vi "Autonomous Independent.vi"() -> ()   [LabVIEW 2015]
doc: "This VI is called when autonomous begins, and will automatically be terminated when autonomous ends. You can carry out timed or sensor driven robot movement independently without needing to return to the caller."
uses:
  Robot Global Data.vi
  <vilib>/Rock Robotics/Network Tables/NT Read Number.vi
panel:
  out "Speed":dbl
  out "Stuck?":bool
  out "Position":dbl
  out "Temporary Center":dbl
  # "Be sure to right-click and choose Data Operations>>Make Current Value default if you want to save the array values with the VI"
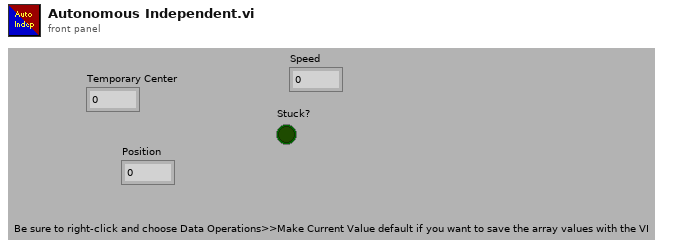
[diagram p1: front panel]
types:
  T1 = typedef "Relevant Data.ctl" = cluster{"Area":dbl, "CH Area":dbl, "BR Width":dbl, "BR Height":dbl, "BR Left":dbl, "BR Right":dbl}
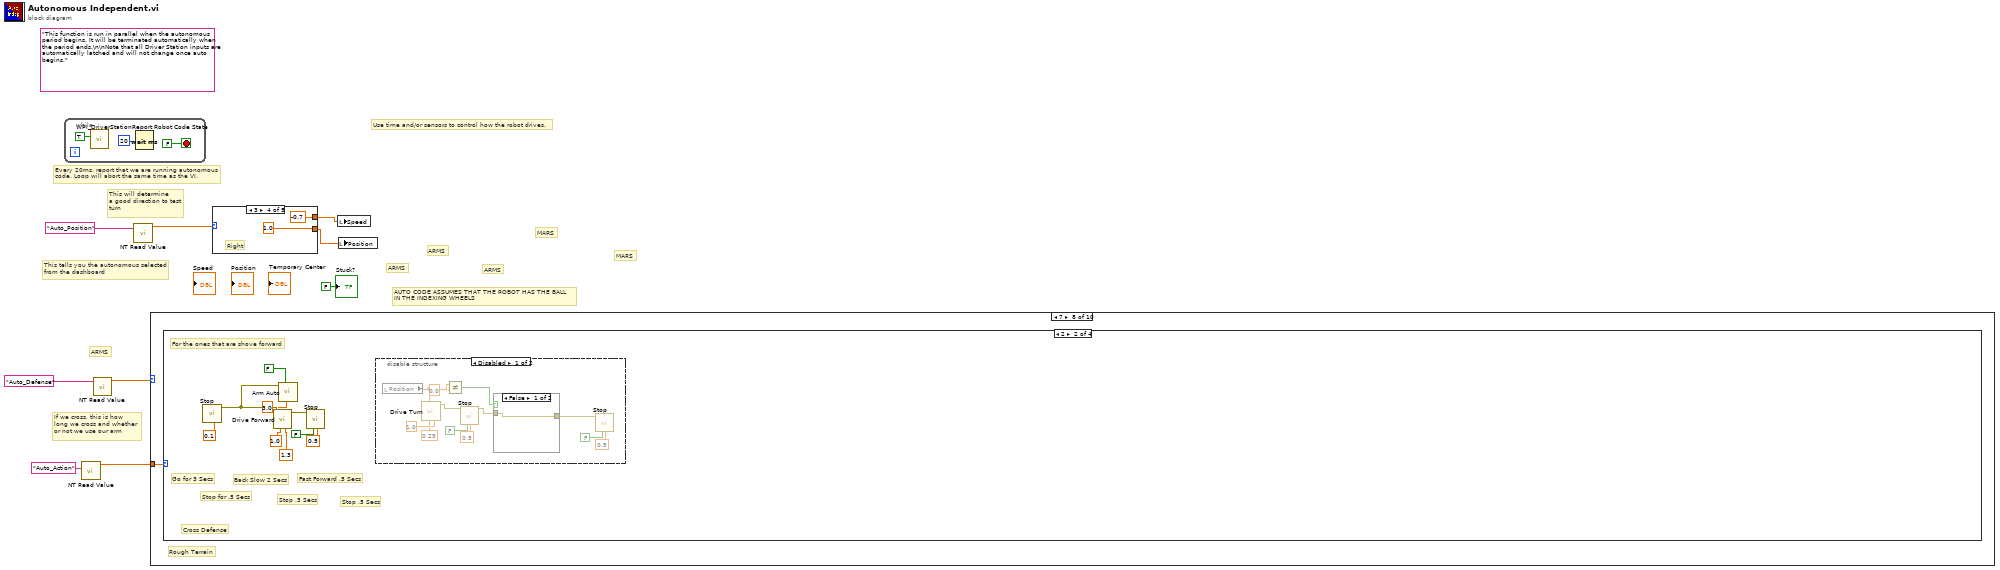
[diagram p0: block diagram]
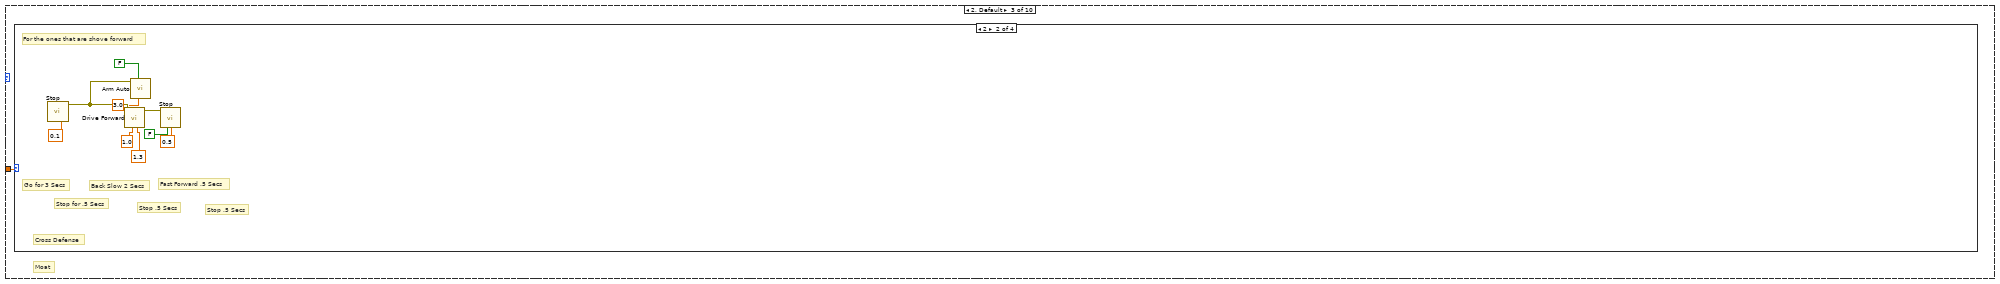
[diagram p4: hidden frame]
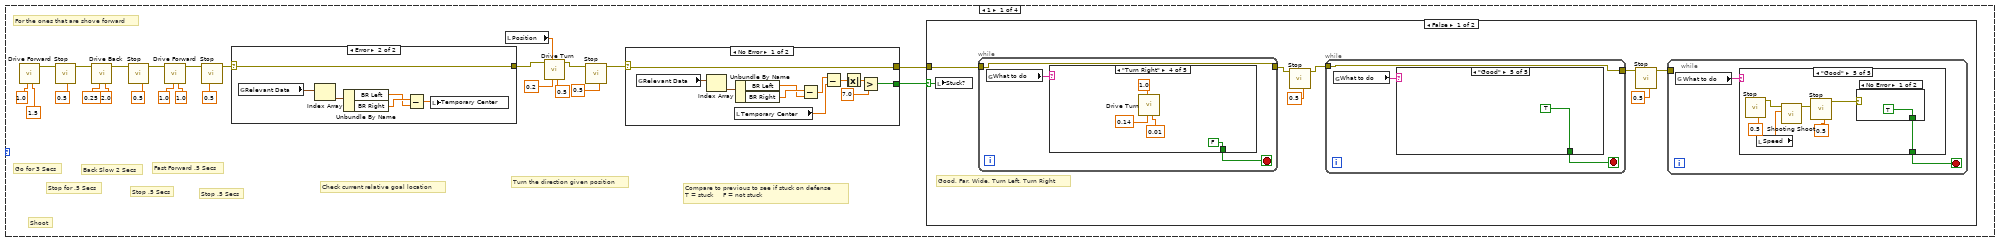
[diagram p5: hidden frame]
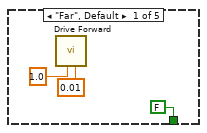
[diagram p6: hidden frame]
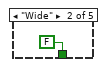
[diagram p7: hidden frame]
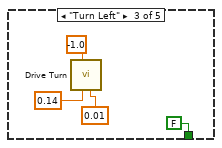
[diagram p8: hidden frame]
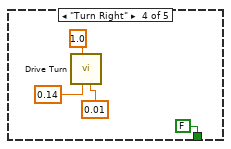
[diagram p9: hidden frame]
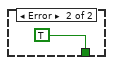
[diagram p10: hidden frame]
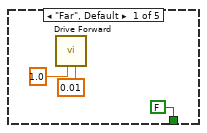
[diagram p11: hidden frame]
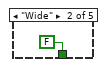
[diagram p12: hidden frame]
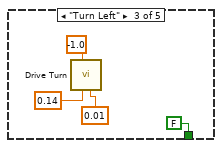
[diagram p13: hidden frame]
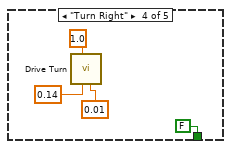
[diagram p14: hidden frame]
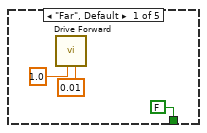
[diagram p15: hidden frame]
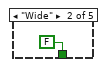
[diagram p16: hidden frame]
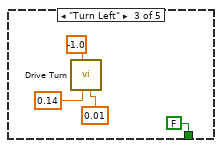
[diagram p17: hidden frame]
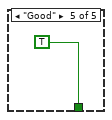
[diagram p18: hidden frame]
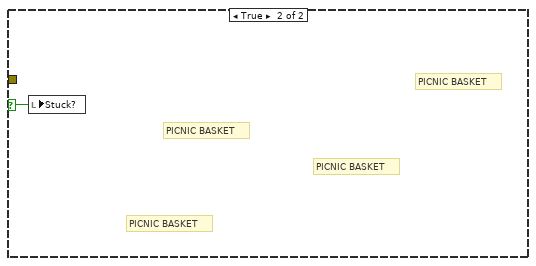
[diagram p19: hidden frame]
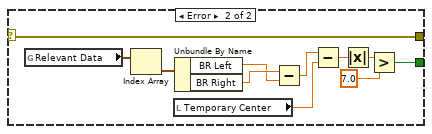
[diagram p20: hidden frame]
diagram:
  (unwired) "This function is run in parallel when the autonomous period begins. It will be terminated automatically when the period ends.\n\nNote that all Driver Station inputs are automatically latched and will not change once auto begins."
  # "MARS"
  # "MARS"
  # "ARMS"
  # "ARMS"
  # "ARMS"
  # "ARMS"
  # "AUTO CODE ASSUMES THAT THE ROBOT HAS THE BALL\nIN THE INDEXING WHEELS"
  # "If we cross, this is how\nlong we cross and whether \nor not we use our arm"
  # "This will determine\na good direction to test\nturn"
  # "This tells you the autonomous selected\nfrom the dashboard"
  # "Every 20ms, report that we are running autonomous\ncode. Loop will abort the same time as the VI."
  # "Use time and/or sensors to control how the robot drives."
  n1 = while {
    stop <- FALSE stop-if-true
    n2 = call <vilib>:"WPI_DriverStationReport Robot Code State.vi"("Autonomous"=TRUE) -> ()  [unwired: 10 in, 1 out]
    n3 = Wait (ms)(milliseconds to wait=u32 20) -> ()  [unwired: 1 out]
  }
  n4 = call-poly <vilib>:"NT Read Value.vi"("Name"="Auto_Action") -> ("Numeric"=w2:dbl)  [unwired: 9 in, 1 out]
  n5 = call-poly <vilib>:"NT Read Value.vi"("Name"="Auto_Defense") -> ("Numeric"=w7:dbl)  [unwired: 9 in, 1 out]
  n6 = call-poly <vilib>:"NT Read Value.vi"("Name"="Auto_Position") -> ("Numeric"=w8:dbl)  [unwired: 9 in, 1 out]
  n7 = case shown="7" w7 {
    tunnel: w2 -> [_ _ w13 w150 _ _ w287 w424 _ w579]
    frame 0 {
      # "Portcullis"
    }
    frame 1 {
      # "Cheval de Frise"
    }
    frame 2, Default {
      # "Moat"
      n8 = case shown="2" w13 {
        frame 1 {
          # "Shoot"
          # "Check current relative goal location"
          # "Stop .5 Secs"
          # "Turn the direction given position"
          # "Compare to previous to see if stuck on defense\nT = stuck     F = not stuck"
          # "Fast Forward .5 Secs"
          # "Stop .5 Secs"
          # "Back Slow 2 Secs"
          # "Stop for .5 Secs"
          # "Go for 3 Secs"
          # "For the ones that are shove forward"
          n9 = call "Drive Forward.vi"("Time"=1.5, "Speed"=1.0) -> ("error out"=w37:errorcluster)  [unwired: 9 in]
          n10 = call "Stop.vi"("Time"=0.5, "error in"=w37) -> ("error out"=w36:errorcluster)  [unwired: 8 in, 1 out]
          n11 = call "Drive Back.vi"("Time"=2.0, "Speed"=0.25, "error in"=w36) -> ("error out"=w35:errorcluster)  [unwired: 8 in]
          n12 = call "Stop.vi"("Time"=0.5, "error in"=w35) -> ("error out"=w34:errorcluster)  [unwired: 8 in, 1 out]
          n13 = call "Drive Forward.vi"("Time"=1.0, "Speed"=1.0, "error in"=w34) -> ("error out"=w33:errorcluster)  [unwired: 8 in]
          n14 = call "Stop.vi"("Time"=0.5, "error in"=w33) -> ("error out"=w23:errorcluster)  [unwired: 8 in, 1 out]
          n15 = case shown="Error" w23 {
            selector: w23 -> [w124 w130]
            tunnel: [w124 w130] -> w22
            frame No Error {
              n16 = global read "Robot Global Data.vi" "Relevant Data"() -> (w129:T1[])
              n17 = Index Array(array=w129) -> (element=w128:T1)  [unwired: 1 in]
              n18 = Unbundle By Name(w128) -> ("BR Left"=w126:dbl, "BR Right"=w127:dbl)
              n19 = Subtract(x=w127, y=w126) -> (x-y=w125:dbl)
              n20 = local write "Temporary Center"(w125) -> ()
            }
            frame Error {
              n21 = global read "Robot Global Data.vi" "Relevant Data"() -> (w135:T1[])
              n22 = Index Array(array=w135) -> (element=w134:T1)  [unwired: 1 in]
              n23 = Unbundle By Name(w134) -> ("BR Left"=w132:dbl, "BR Right"=w133:dbl)
              n24 = Subtract(x=w133, y=w132) -> (x-y=w131:dbl)
              n25 = local write "Temporary Center"(w131) -> ()
            }
          }
          n26 = local read "Position"() -> (w21:dbl)
          n27 = call "Drive Turn.vi"("Time"=0.5, "Speed"=0.2, "Direction"=w21, "error in"=w22) -> ("error out"=w17:errorcluster)  [unwired: 7 in]
          n28 = call "Stop.vi"("Time"=0.5, "error in"=w17) -> ("error out"=w16:errorcluster)  [unwired: 8 in, 1 out]
          n29 = case shown="No Error" w16 {
            selector: w16 -> [w108 w119]
            tunnel: [w108 w119] -> w14
            tunnel: [w102 w113] -> w18
            frame No Error {
              n30 = global read "Robot Global Data.vi" "Relevant Data"() -> (w112:T1[])
              n31 = Index Array(array=w112) -> (element=w111:T1)  [unwired: 1 in]
              n32 = local read "Temporary Center"() -> (w106:dbl)
              n33 = Unbundle By Name(w111) -> ("BR Left"=w109:dbl, "BR Right"=w110:dbl)
              n34 = Subtract(x=w110, y=w109) -> (x-y=w107:dbl)
              n35 = Subtract(x=w107, y=w106) -> (x-y=w105:dbl)
              n36 = Absolute Value(x=w105) -> (abs(x)=w104:dbl)
              n37 = Greater?(x=w104, y=7.0) -> (0:w102:bool)
            }
            frame Error {
              n38 = global read "Robot Global Data.vi" "Relevant Data"() -> (w123:T1[])
              n39 = Index Array(array=w123) -> (element=w122:T1)  [unwired: 1 in]
              n40 = local read "Temporary Center"() -> (w117:dbl)
              n41 = Unbundle By Name(w122) -> ("BR Left"=w120:dbl, "BR Right"=w121:dbl)
              n42 = Subtract(x=w121, y=w120) -> (x-y=w118:dbl)
              n43 = Subtract(x=w118, y=w117) -> (x-y=w116:dbl)
              n44 = Absolute Value(x=w116) -> (abs(x)=w115:dbl)
              n45 = Greater?(x=w115, y=7.0) -> (0:w113:bool)
            }
          }
          n46 = case shown="False" w18 {
            selector: w18 -> [w45 w101]
            tunnel: w14 -> [w44 _]
            frame False {
              # "Good, Far, Wide, Turn Left, Turn Right"
              n47 = local write "Stuck?"(w45) -> ()
              n48 = while {
                tunnel: w44 -> [w85]
                tunnel: [w85] -> w43
                stop <- w86 stop-if-true
                n49 = global read "Robot Global Data.vi" "What to do"() -> (w87:string)
                n50 = case shown="\"Turn Right\"" w87 {
                  tunnel: [FALSE FALSE FALSE FALSE TRUE] -> w86
                  frame "Far", Default {
                    n51 = call "Drive Forward.vi"("Time"=0.01, "Speed"=1.0) -> ()  [unwired: 9 in, 1 out]
                  }
                  frame "Wide" {
                  }
                  frame "Turn Left" {
                    n52 = call "Drive Turn.vi"("Time"=0.01, "Speed"=0.14, "Direction"=-1.0) -> ()  [unwired: 8 in, 1 out]
                  }
                  frame "Turn Right" {
                    n53 = call "Drive Turn.vi"("Time"=0.01, "Speed"=0.14, "Direction"=1.0) -> ()  [unwired: 8 in, 1 out]
                  }
                  frame "Good" {
                  }
                }
              }
              n54 = call "Stop.vi"("Time"=0.5, "error in"=w43) -> ("error out"=w42:errorcluster)  [unwired: 8 in, 1 out]
              n55 = while {
                tunnel: w42 -> [w69]
                tunnel: [w69] -> w40
                stop <- w70 stop-if-true
                n56 = global read "Robot Global Data.vi" "What to do"() -> (w71:string)
                n57 = case shown="\"Good\"" w71 {
                  tunnel: [FALSE FALSE FALSE FALSE TRUE] -> w70
                  frame "Far", Default {
                    n58 = call "Drive Forward.vi"("Time"=0.01, "Speed"=1.0) -> ()  [unwired: 9 in, 1 out]
                  }
                  frame "Wide" {
                  }
                  frame "Turn Left" {
                    n59 = call "Drive Turn.vi"("Time"=0.01, "Speed"=0.14, "Direction"=-1.0) -> ()  [unwired: 8 in, 1 out]
                  }
                  frame "Turn Right" {
                    n60 = call "Drive Turn.vi"("Time"=0.01, "Speed"=0.14, "Direction"=1.0) -> ()  [unwired: 8 in, 1 out]
                  }
                  frame "Good" {
                  }
                }
              }
              n61 = call "Stop.vi"("Time"=0.5, "error in"=w40) -> ("error out"=w39:errorcluster)  [unwired: 8 in, 1 out]
              n62 = while {
                tunnel: w39 -> [_]
                stop <- w46 stop-if-true
                n63 = global read "Robot Global Data.vi" "What to do"() -> (w47:string)
                n64 = case shown="\"Good\"" w47 {
                  tunnel: [FALSE FALSE FALSE FALSE w64] -> w46
                  frame "Far", Default {
                    n65 = call "Drive Forward.vi"("Time"=0.01, "Speed"=1.0) -> ()  [unwired: 9 in, 1 out]
                  }
                  frame "Wide" {
                  }
                  frame "Turn Left" {
                    n66 = call "Drive Turn.vi"("Time"=0.01, "Speed"=0.14, "Direction"=-1.0) -> ()  [unwired: 8 in, 1 out]
                  }
                  frame "Turn Right" {
                    n67 = call "Drive Turn.vi"("Time"=0.01, "Speed"=0.14, "Direction"=1.0) -> ()  [unwired: 8 in, 1 out]
                  }
                  frame "Good" {
                    n68 = call "Stop.vi"("Time"=0.5) -> ("error out"=w61:errorcluster)  [unwired: 9 in, 1 out]
                    n69 = local read "Speed"() -> (w60:dbl)
                    n70 = call "Shooting Shoot.vi"("Power"=w60, "error in (no error)"=w61) -> ("error out"=w62:errorcluster)  [unwired: 9 in]
                    n71 = call "Stop.vi"("Time"=0.5, "error in"=w62) -> ("error out"=w65:errorcluster)  [unwired: 8 in, 1 out]
                    n72 = case shown="No Error" w65 {
                      tunnel: [TRUE TRUE] -> w64
                      frame No Error {
                      }
                      frame Error {
                      }
                    }
                  }
                }
              }
            }
            frame True {
              # "PICNIC BASKET"
              # "PICNIC BASKET"
              # "PICNIC BASKET"
              # "PICNIC BASKET"
              n73 = local write "Stuck?"(w101) -> ()
            }
          }
        }
        frame 2 {
          # "Cross Defense"
          # "Stop .5 Secs"
          # "Fast Forward .5 Secs"
          # "Stop .5 Secs"
          # "Back Slow 2 Secs"
          # "Stop for .5 Secs"
          # "Go for 3 Secs"
          # "For the ones that are shove forward"
          n74 = call "Stop.vi"("Time"=0.1) -> ("error out"=w139:errorcluster)  [unwired: 9 in, 1 out]
          n75 = call "Drive Forward.vi"("Time"=1.3, "Speed"=1.0, "error in"=w139) -> ("error out"=w144:errorcluster)  [unwired: 8 in]
          n76 = call "Arm Auto.vi"("Time"=3.0, "U=T\nD=F"=FALSE ("U=T\nD=F"), "error in"=w139) -> ()  [unwired: 8 in, 1 out]
          n77 = call "Stop.vi"("Time"=0.5, "Stop Arm?"=FALSE, "error in"=w144) -> ()  [unwired: 7 in, 2 out]
        }
        frame 3 {
          # "Up to Line"
          # "Stop for .5 Secs"
          # "Go for 3 Secs"
          # "For the ones that are shove forward"
          n78 = call "Drive Forward.vi"("Time"=0.5, "Speed"=1.0) -> ("error out"=w148:errorcluster)  [unwired: 9 in]
          n79 = call "Stop.vi"("Time"=0.5, "error in"=w148) -> ()  [unwired: 8 in, 2 out]
        }
        frame 0, Default {
          # "Disabled"
          n80 = call "Stop.vi"("Time"=0.5) -> ()  [unwired: 9 in, 2 out]
        }
      }
    }
    frame 3 {
      # "Ramparts"
      n81 = case shown="2" w150 {
        frame 1 {
          # "Shoot"
          # "Check current relative goal location"
          # "Stop .5 Secs"
          # "Turn the direction given position"
          # "Compare to previous to see if stuck on defense\nT = stuck     F = not stuck"
          # "Fast Forward .5 Secs"
          # "Stop .5 Secs"
          # "Back Slow 2 Secs"
          # "Stop for .5 Secs"
          # "Go for 3 Secs"
          # "For the ones that are shove forward"
          n82 = call "Drive Forward.vi"("Time"=1.5, "Speed"=1.0) -> ("error out"=w174:errorcluster)  [unwired: 9 in]
          n83 = call "Stop.vi"("Time"=0.5, "error in"=w174) -> ("error out"=w173:errorcluster)  [unwired: 8 in, 1 out]
          n84 = call "Drive Back.vi"("Time"=2.0, "Speed"=0.25, "error in"=w173) -> ("error out"=w172:errorcluster)  [unwired: 8 in]
          n85 = call "Stop.vi"("Time"=0.5, "error in"=w172) -> ("error out"=w171:errorcluster)  [unwired: 8 in, 1 out]
          n86 = call "Drive Forward.vi"("Time"=1.0, "Speed"=1.0, "error in"=w171) -> ("error out"=w170:errorcluster)  [unwired: 8 in]
          n87 = call "Stop.vi"("Time"=0.5, "error in"=w170) -> ("error out"=w160:errorcluster)  [unwired: 8 in, 1 out]
          n88 = case shown="Error" w160 {
            selector: w160 -> [w261 w267]
            tunnel: [w261 w267] -> w159
            frame No Error {
              n89 = global read "Robot Global Data.vi" "Relevant Data"() -> (w266:T1[])
              n90 = Index Array(array=w266) -> (element=w265:T1)  [unwired: 1 in]
              n91 = Unbundle By Name(w265) -> ("BR Left"=w263:dbl, "BR Right"=w264:dbl)
              n92 = Subtract(x=w264, y=w263) -> (x-y=w262:dbl)
              n93 = local write "Temporary Center"(w262) -> ()
            }
            frame Error {
              n94 = global read "Robot Global Data.vi" "Relevant Data"() -> (w272:T1[])
              n95 = Index Array(array=w272) -> (element=w271:T1)  [unwired: 1 in]
              n96 = Unbundle By Name(w271) -> ("BR Left"=w269:dbl, "BR Right"=w270:dbl)
              n97 = Subtract(x=w270, y=w269) -> (x-y=w268:dbl)
              n98 = local write "Temporary Center"(w268) -> ()
            }
          }
          n99 = call "Drive Turn.vi"("Time"=0.5, "Speed"=0.2, "Direction"=-1.0, "error in"=w159) -> ("error out"=w155:errorcluster)  [unwired: 7 in]
          n100 = call "Stop.vi"("Time"=0.5, "error in"=w155) -> ("error out"=w154:errorcluster)  [unwired: 8 in, 1 out]
          n101 = case shown="No Error" w154 {
            selector: w154 -> [w245 w256]
            tunnel: [w245 w256] -> w152
            tunnel: [w239 w250] -> w156
            frame No Error {
              n102 = global read "Robot Global Data.vi" "Relevant Data"() -> (w249:T1[])
              n103 = Index Array(array=w249) -> (element=w248:T1)  [unwired: 1 in]
              n104 = local read "Temporary Center"() -> (w243:dbl)
              n105 = Unbundle By Name(w248) -> ("BR Left"=w246:dbl, "BR Right"=w247:dbl)
              n106 = Subtract(x=w247, y=w246) -> (x-y=w244:dbl)
              n107 = Subtract(x=w244, y=w243) -> (x-y=w242:dbl)
              n108 = Absolute Value(x=w242) -> (abs(x)=w241:dbl)
              n109 = Greater?(x=w241, y=7.0) -> (0:w239:bool)
            }
            frame Error {
              n110 = global read "Robot Global Data.vi" "Relevant Data"() -> (w260:T1[])
              n111 = Index Array(array=w260) -> (element=w259:T1)  [unwired: 1 in]
              n112 = local read "Temporary Center"() -> (w254:dbl)
              n113 = Unbundle By Name(w259) -> ("BR Left"=w257:dbl, "BR Right"=w258:dbl)
              n114 = Subtract(x=w258, y=w257) -> (x-y=w255:dbl)
              n115 = Subtract(x=w255, y=w254) -> (x-y=w253:dbl)
              n116 = Absolute Value(x=w253) -> (abs(x)=w252:dbl)
              n117 = Greater?(x=w252, y=7.0) -> (0:w250:bool)
            }
          }
          n118 = case shown="False" w156 {
            selector: w156 -> [w182 w238]
            tunnel: w152 -> [w181 _]
            frame False {
              # "Good, Far, Wide, Turn Left, Turn Right"
              n119 = local write "Stuck?"(w182) -> ()
              n120 = while {
                tunnel: w181 -> [w222]
                tunnel: [w222] -> w180
                stop <- w223 stop-if-true
                n121 = global read "Robot Global Data.vi" "What to do"() -> (w224:string)
                n122 = case shown="\"Turn Right\"" w224 {
                  tunnel: [FALSE FALSE FALSE FALSE TRUE] -> w223
                  frame "Far", Default {
                    n123 = call "Drive Forward.vi"("Time"=0.01, "Speed"=1.0) -> ()  [unwired: 9 in, 1 out]
                  }
                  frame "Wide" {
                  }
                  frame "Turn Left" {
                    n124 = call "Drive Turn.vi"("Time"=0.01, "Speed"=0.14, "Direction"=-1.0) -> ()  [unwired: 8 in, 1 out]
                  }
                  frame "Turn Right" {
                    n125 = call "Drive Turn.vi"("Time"=0.01, "Speed"=0.14, "Direction"=1.0) -> ()  [unwired: 8 in, 1 out]
                  }
                  frame "Good" {
                  }
                }
              }
              n126 = call "Stop.vi"("Time"=0.5, "error in"=w180) -> ("error out"=w179:errorcluster)  [unwired: 8 in, 1 out]
              n127 = while {
                tunnel: w179 -> [w206]
                tunnel: [w206] -> w177
                stop <- w207 stop-if-true
                n128 = global read "Robot Global Data.vi" "What to do"() -> (w208:string)
                n129 = case shown="\"Good\"" w208 {
                  tunnel: [FALSE FALSE FALSE FALSE TRUE] -> w207
                  frame "Far", Default {
                    n130 = call "Drive Forward.vi"("Time"=0.01, "Speed"=1.0) -> ()  [unwired: 9 in, 1 out]
                  }
                  frame "Wide" {
                  }
                  frame "Turn Left" {
                    n131 = call "Drive Turn.vi"("Time"=0.01, "Speed"=0.14, "Direction"=-1.0) -> ()  [unwired: 8 in, 1 out]
                  }
                  frame "Turn Right" {
                    n132 = call "Drive Turn.vi"("Time"=0.01, "Speed"=0.14, "Direction"=1.0) -> ()  [unwired: 8 in, 1 out]
                  }
                  frame "Good" {
                  }
                }
              }
              n133 = call "Stop.vi"("Time"=0.5, "error in"=w177) -> ("error out"=w176:errorcluster)  [unwired: 8 in, 1 out]
              n134 = while {
                tunnel: w176 -> [_]
                stop <- w183 stop-if-true
                n135 = global read "Robot Global Data.vi" "What to do"() -> (w184:string)
                n136 = case shown="\"Good\"" w184 {
                  tunnel: [FALSE FALSE FALSE FALSE w201] -> w183
                  frame "Far", Default {
                    n137 = call "Drive Forward.vi"("Time"=0.01, "Speed"=1.0) -> ()  [unwired: 9 in, 1 out]
                  }
                  frame "Wide" {
                  }
                  frame "Turn Left" {
                    n138 = call "Drive Turn.vi"("Time"=0.01, "Speed"=0.14, "Direction"=-1.0) -> ()  [unwired: 8 in, 1 out]
                  }
                  frame "Turn Right" {
                    n139 = call "Drive Turn.vi"("Time"=0.01, "Speed"=0.14, "Direction"=1.0) -> ()  [unwired: 8 in, 1 out]
                  }
                  frame "Good" {
                    n140 = call "Stop.vi"("Time"=0.5) -> ("error out"=w198:errorcluster)  [unwired: 9 in, 1 out]
                    n141 = local read "Speed"() -> (w197:dbl)
                    n142 = call "Shooting Shoot.vi"("Power"=w197, "error in (no error)"=w198) -> ("error out"=w199:errorcluster)  [unwired: 9 in]
                    n143 = call "Stop.vi"("Time"=0.5, "error in"=w199) -> ("error out"=w202:errorcluster)  [unwired: 8 in, 1 out]
                    n144 = case shown="No Error" w202 {
                      tunnel: [TRUE TRUE] -> w201
                      frame No Error {
                      }
                      frame Error {
                      }
                    }
                  }
                }
              }
            }
            frame True {
              # "PICNIC BASKET"
              # "PICNIC BASKET"
              # "PICNIC BASKET"
              # "PICNIC BASKET"
              n145 = local write "Stuck?"(w238) -> ()
            }
          }
        }
        frame 2 {
          # "Cross Defense"
          # "Stop .5 Secs"
          # "Fast Forward .5 Secs"
          # "Stop .5 Secs"
          # "Back Slow 2 Secs"
          # "Stop for .5 Secs"
          # "Go for 3 Secs"
          # "For the ones that are shove forward"
          n146 = call "Stop.vi"("Time"=0.1) -> ("error out"=w274:errorcluster)  [unwired: 9 in, 1 out]
          n147 = call "Drive Forward.vi"("Time"=1.3, "Speed"=1.0, "error in"=w274) -> ("error out"=w279:errorcluster)  [unwired: 8 in]
          n148 = call "Stop.vi"("Time"=0.5, "Stop Arm?"=FALSE, "error in"=w279) -> ()  [unwired: 7 in, 2 out]
        }
        frame 3 {
          # "Up to Line"
          # "Stop for .5 Secs"
          # "Go for 3 Secs"
          # "For the ones that are shove forward"
          n149 = call "Drive Forward.vi"("Time"=0.5, "Speed"=1.0) -> ("error out"=w283:errorcluster)  [unwired: 9 in]
          n150 = call "Stop.vi"("Time"=0.5, "error in"=w283) -> ()  [unwired: 8 in, 2 out]
        }
        frame 0, Default {
          # "Disabled"
          n151 = call "Stop.vi"("Time"=0.5) -> ()  [unwired: 9 in, 2 out]
        }
      }
    }
    frame 4 {
      # "Drawbridge"
      n152 = call "Stop.vi"("Time"=0.5) -> ()  [unwired: 9 in, 2 out]
    }
    frame 5 {
      # "Sally Port"
      n153 = call "Stop.vi"("Time"=0.5) -> ()  [unwired: 9 in, 2 out]
    }
    frame 6 {
      # "Rock Wall"
      n154 = case shown="2" w287 {
        frame 1 {
          # "Shoot"
          # "Check current relative goal location"
          # "Stop .5 Secs"
          # "Turn the direction given position"
          # "Compare to previous to see if stuck on defense\nT = stuck     F = not stuck"
          # "Fast Forward .5 Secs"
          # "Stop .5 Secs"
          # "Back Slow 2 Secs"
          # "Stop for .5 Secs"
          # "Go for 3 Secs"
          # "For the ones that are shove forward"
          n155 = call "Drive Forward.vi"("Time"=1.5, "Speed"=1.0) -> ("error out"=w311:errorcluster)  [unwired: 9 in]
          n156 = call "Stop.vi"("Time"=0.5, "error in"=w311) -> ("error out"=w310:errorcluster)  [unwired: 8 in, 1 out]
          n157 = call "Drive Back.vi"("Time"=2.0, "Speed"=0.25, "error in"=w310) -> ("error out"=w309:errorcluster)  [unwired: 8 in]
          n158 = call "Stop.vi"("Time"=0.5, "error in"=w309) -> ("error out"=w308:errorcluster)  [unwired: 8 in, 1 out]
          n159 = call "Drive Forward.vi"("Time"=1.0, "Speed"=1.0, "error in"=w308) -> ("error out"=w307:errorcluster)  [unwired: 8 in]
          n160 = call "Stop.vi"("Time"=0.5, "error in"=w307) -> ("error out"=w297:errorcluster)  [unwired: 8 in, 1 out]
          n161 = case shown="Error" w297 {
            selector: w297 -> [w398 w404]
            tunnel: [w398 w404] -> w296
            frame No Error {
              n162 = global read "Robot Global Data.vi" "Relevant Data"() -> (w403:T1[])
              n163 = Index Array(array=w403) -> (element=w402:T1)  [unwired: 1 in]
              n164 = Unbundle By Name(w402) -> ("BR Left"=w400:dbl, "BR Right"=w401:dbl)
              n165 = Subtract(x=w401, y=w400) -> (x-y=w399:dbl)
              n166 = local write "Temporary Center"(w399) -> ()
            }
            frame Error {
              n167 = global read "Robot Global Data.vi" "Relevant Data"() -> (w409:T1[])
              n168 = Index Array(array=w409) -> (element=w408:T1)  [unwired: 1 in]
              n169 = Unbundle By Name(w408) -> ("BR Left"=w406:dbl, "BR Right"=w407:dbl)
              n170 = Subtract(x=w407, y=w406) -> (x-y=w405:dbl)
              n171 = local write "Temporary Center"(w405) -> ()
            }
          }
          n172 = local read "Position"() -> (w295:dbl)
          n173 = call "Drive Turn.vi"("Time"=0.5, "Speed"=0.2, "Direction"=w295, "error in"=w296) -> ("error out"=w291:errorcluster)  [unwired: 7 in]
          n174 = call "Stop.vi"("Time"=0.5, "error in"=w291) -> ("error out"=w290:errorcluster)  [unwired: 8 in, 1 out]
          n175 = case shown="No Error" w290 {
            selector: w290 -> [w382 w393]
            tunnel: [w382 w393] -> w288
            tunnel: [w376 w387] -> w292
            frame No Error {
              n176 = global read "Robot Global Data.vi" "Relevant Data"() -> (w386:T1[])
              n177 = Index Array(array=w386) -> (element=w385:T1)  [unwired: 1 in]
              n178 = local read "Temporary Center"() -> (w380:dbl)
              n179 = Unbundle By Name(w385) -> ("BR Left"=w383:dbl, "BR Right"=w384:dbl)
              n180 = Subtract(x=w384, y=w383) -> (x-y=w381:dbl)
              n181 = Subtract(x=w381, y=w380) -> (x-y=w379:dbl)
              n182 = Absolute Value(x=w379) -> (abs(x)=w378:dbl)
              n183 = Greater?(x=w378, y=7.0) -> (0:w376:bool)
            }
            frame Error {
              n184 = global read "Robot Global Data.vi" "Relevant Data"() -> (w397:T1[])
              n185 = Index Array(array=w397) -> (element=w396:T1)  [unwired: 1 in]
              n186 = local read "Temporary Center"() -> (w391:dbl)
              n187 = Unbundle By Name(w396) -> ("BR Left"=w394:dbl, "BR Right"=w395:dbl)
              n188 = Subtract(x=w395, y=w394) -> (x-y=w392:dbl)
              n189 = Subtract(x=w392, y=w391) -> (x-y=w390:dbl)
              n190 = Absolute Value(x=w390) -> (abs(x)=w389:dbl)
              n191 = Greater?(x=w389, y=7.0) -> (0:w387:bool)
            }
          }
          n192 = case shown="False" w292 {
            selector: w292 -> [w319 w375]
            tunnel: w288 -> [w318 _]
            frame False {
              # "Good, Far, Wide, Turn Left, Turn Right"
              n193 = local write "Stuck?"(w319) -> ()
              n194 = while {
                tunnel: w318 -> [w359]
                tunnel: [w359] -> w317
                stop <- w360 stop-if-true
                n195 = global read "Robot Global Data.vi" "What to do"() -> (w361:string)
                n196 = case shown="\"Turn Right\"" w361 {
                  tunnel: [FALSE FALSE FALSE FALSE TRUE] -> w360
                  frame "Far", Default {
                    n197 = call "Drive Forward.vi"("Time"=0.01, "Speed"=1.0) -> ()  [unwired: 9 in, 1 out]
                  }
                  frame "Wide" {
                  }
                  frame "Turn Left" {
                    n198 = call "Drive Turn.vi"("Time"=0.01, "Speed"=0.14, "Direction"=-1.0) -> ()  [unwired: 8 in, 1 out]
                  }
                  frame "Turn Right" {
                    n199 = call "Drive Turn.vi"("Time"=0.01, "Speed"=0.14, "Direction"=1.0) -> ()  [unwired: 8 in, 1 out]
                  }
                  frame "Good" {
                  }
                }
              }
              n200 = call "Stop.vi"("Time"=0.5, "error in"=w317) -> ("error out"=w316:errorcluster)  [unwired: 8 in, 1 out]
              n201 = while {
                tunnel: w316 -> [w343]
                tunnel: [w343] -> w314
                stop <- w344 stop-if-true
                n202 = global read "Robot Global Data.vi" "What to do"() -> (w345:string)
                n203 = case shown="\"Good\"" w345 {
                  tunnel: [FALSE FALSE FALSE FALSE TRUE] -> w344
                  frame "Far", Default {
                    n204 = call "Drive Forward.vi"("Time"=0.01, "Speed"=1.0) -> ()  [unwired: 9 in, 1 out]
                  }
                  frame "Wide" {
                  }
                  frame "Turn Left" {
                    n205 = call "Drive Turn.vi"("Time"=0.01, "Speed"=0.14, "Direction"=-1.0) -> ()  [unwired: 8 in, 1 out]
                  }
                  frame "Turn Right" {
                    n206 = call "Drive Turn.vi"("Time"=0.01, "Speed"=0.14, "Direction"=1.0) -> ()  [unwired: 8 in, 1 out]
                  }
                  frame "Good" {
                  }
                }
              }
              n207 = call "Stop.vi"("Time"=0.5, "error in"=w314) -> ("error out"=w313:errorcluster)  [unwired: 8 in, 1 out]
              n208 = while {
                tunnel: w313 -> [_]
                stop <- w320 stop-if-true
                n209 = global read "Robot Global Data.vi" "What to do"() -> (w321:string)
                n210 = case shown="\"Good\"" w321 {
                  tunnel: [FALSE FALSE FALSE FALSE w338] -> w320
                  frame "Far", Default {
                    n211 = call "Drive Forward.vi"("Time"=0.01, "Speed"=1.0) -> ()  [unwired: 9 in, 1 out]
                  }
                  frame "Wide" {
                  }
                  frame "Turn Left" {
                    n212 = call "Drive Turn.vi"("Time"=0.01, "Speed"=0.14, "Direction"=-1.0) -> ()  [unwired: 8 in, 1 out]
                  }
                  frame "Turn Right" {
                    n213 = call "Drive Turn.vi"("Time"=0.01, "Speed"=0.14, "Direction"=1.0) -> ()  [unwired: 8 in, 1 out]
                  }
                  frame "Good" {
                    n214 = call "Stop.vi"("Time"=0.5) -> ("error out"=w335:errorcluster)  [unwired: 9 in, 1 out]
                    n215 = local read "Speed"() -> (w334:dbl)
                    n216 = call "Shooting Shoot.vi"("Power"=w334, "error in (no error)"=w335) -> ("error out"=w336:errorcluster)  [unwired: 9 in]
                    n217 = call "Stop.vi"("Time"=0.5, "error in"=w336) -> ("error out"=w339:errorcluster)  [unwired: 8 in, 1 out]
                    n218 = case shown="No Error" w339 {
                      tunnel: [TRUE TRUE] -> w338
                      frame No Error {
                      }
                      frame Error {
                      }
                    }
                  }
                }
              }
            }
            frame True {
              # "PICNIC BASKET"
              # "PICNIC BASKET"
              # "PICNIC BASKET"
              # "PICNIC BASKET"
              n219 = local write "Stuck?"(w375) -> ()
            }
          }
        }
        frame 2 {
          # "Cross Defense"
          # "Stop .5 Secs"
          # "Fast Forward .5 Secs"
          # "Stop .5 Secs"
          # "Back Slow 2 Secs"
          # "Stop for .5 Secs"
          # "Go for 3 Secs"
          # "For the ones that are shove forward"
          n220 = call "Stop.vi"("Time"=0.1) -> ("error out"=w413:errorcluster)  [unwired: 9 in, 1 out]
          n221 = call "Drive Forward.vi"("Time"=1.3, "Speed"=1.0, "error in"=w413) -> ("error out"=w418:errorcluster)  [unwired: 8 in]
          n222 = call "Arm Auto.vi"("Time"=3.0, "U=T\nD=F"=FALSE ("U=T\nD=F"), "error in"=w413) -> ()  [unwired: 8 in, 1 out]
          n223 = call "Stop.vi"("Time"=0.5, "Stop Arm?"=FALSE, "error in"=w418) -> ()  [unwired: 7 in, 2 out]
        }
        frame 3 {
          # "Up to Line"
          # "Stop for .5 Secs"
          # "Go for 3 Secs"
          # "For the ones that are shove forward"
          n224 = call "Drive Forward.vi"("Time"=0.5, "Speed"=1.0) -> ("error out"=w422:errorcluster)  [unwired: 9 in]
          n225 = call "Stop.vi"("Time"=0.5, "error in"=w422) -> ()  [unwired: 8 in, 2 out]
        }
        frame 0, Default {
          # "Disabled"
          n226 = call "Stop.vi"("Time"=0.5) -> ()  [unwired: 9 in, 2 out]
        }
      }
    }
    frame 7 {
      # "Rough Terrain"
      n227 = case shown="2" w424 {
        frame 1 {
          # "Shoot"
          # "Check current relative goal location"
          # "Stop .5 Secs"
          # "Turn the direction given position"
          # "Compare to previous to see if stuck on defense\nT = stuck     F = not stuck"
          # "Fast Forward .5 Secs"
          # "Stop .5 Secs"
          # "Back Slow 2 Secs"
          # "Stop for .5 Secs"
          # "Go for 3 Secs"
          # "For the ones that are shove forward"
          n228 = call "Drive Forward.vi"("Time"=1.5, "Speed"=1.0) -> ("error out"=w448:errorcluster)  [unwired: 9 in]
          n229 = call "Stop.vi"("Time"=0.5, "error in"=w448) -> ("error out"=w447:errorcluster)  [unwired: 8 in, 1 out]
          n230 = call "Drive Back.vi"("Time"=2.0, "Speed"=0.25, "error in"=w447) -> ("error out"=w446:errorcluster)  [unwired: 8 in]
          n231 = call "Stop.vi"("Time"=0.5, "error in"=w446) -> ("error out"=w445:errorcluster)  [unwired: 8 in, 1 out]
          n232 = call "Drive Forward.vi"("Time"=1.0, "Speed"=1.0, "error in"=w445) -> ("error out"=w444:errorcluster)  [unwired: 8 in]
          n233 = call "Stop.vi"("Time"=0.5, "error in"=w444) -> ("error out"=w434:errorcluster)  [unwired: 8 in, 1 out]
          n234 = case shown="Error" w434 {
            selector: w434 -> [w535 w541]
            tunnel: [w535 w541] -> w433
            frame No Error {
              n235 = global read "Robot Global Data.vi" "Relevant Data"() -> (w540:T1[])
              n236 = Index Array(array=w540) -> (element=w539:T1)  [unwired: 1 in]
              n237 = Unbundle By Name(w539) -> ("BR Left"=w537:dbl, "BR Right"=w538:dbl)
              n238 = Subtract(x=w538, y=w537) -> (x-y=w536:dbl)
              n239 = local write "Temporary Center"(w536) -> ()
            }
            frame Error {
              n240 = global read "Robot Global Data.vi" "Relevant Data"() -> (w546:T1[])
              n241 = Index Array(array=w546) -> (element=w545:T1)  [unwired: 1 in]
              n242 = Unbundle By Name(w545) -> ("BR Left"=w543:dbl, "BR Right"=w544:dbl)
              n243 = Subtract(x=w544, y=w543) -> (x-y=w542:dbl)
              n244 = local write "Temporary Center"(w542) -> ()
            }
          }
          n245 = local read "Position"() -> (w432:dbl)
          n246 = call "Drive Turn.vi"("Time"=0.5, "Speed"=0.2, "Direction"=w432, "error in"=w433) -> ("error out"=w428:errorcluster)  [unwired: 7 in]
          n247 = call "Stop.vi"("Time"=0.5, "error in"=w428) -> ("error out"=w427:errorcluster)  [unwired: 8 in, 1 out]
          n248 = case shown="No Error" w427 {
            selector: w427 -> [w519 w530]
            tunnel: [w519 w530] -> w425
            tunnel: [w513 w524] -> w429
            frame No Error {
              n249 = global read "Robot Global Data.vi" "Relevant Data"() -> (w523:T1[])
              n250 = Index Array(array=w523) -> (element=w522:T1)  [unwired: 1 in]
              n251 = local read "Temporary Center"() -> (w517:dbl)
              n252 = Unbundle By Name(w522) -> ("BR Left"=w520:dbl, "BR Right"=w521:dbl)
              n253 = Subtract(x=w521, y=w520) -> (x-y=w518:dbl)
              n254 = Subtract(x=w518, y=w517) -> (x-y=w516:dbl)
              n255 = Absolute Value(x=w516) -> (abs(x)=w515:dbl)
              n256 = Greater?(x=w515, y=7.0) -> (0:w513:bool)
            }
            frame Error {
              n257 = global read "Robot Global Data.vi" "Relevant Data"() -> (w534:T1[])
              n258 = Index Array(array=w534) -> (element=w533:T1)  [unwired: 1 in]
              n259 = local read "Temporary Center"() -> (w528:dbl)
              n260 = Unbundle By Name(w533) -> ("BR Left"=w531:dbl, "BR Right"=w532:dbl)
              n261 = Subtract(x=w532, y=w531) -> (x-y=w529:dbl)
              n262 = Subtract(x=w529, y=w528) -> (x-y=w527:dbl)
              n263 = Absolute Value(x=w527) -> (abs(x)=w526:dbl)
              n264 = Greater?(x=w526, y=7.0) -> (0:w524:bool)
            }
          }
          n265 = case shown="False" w429 {
            selector: w429 -> [w456 w512]
            tunnel: w425 -> [w455 _]
            frame False {
              # "Good, Far, Wide, Turn Left, Turn Right"
              n266 = local write "Stuck?"(w456) -> ()
              n267 = while {
                tunnel: w455 -> [w496]
                tunnel: [w496] -> w454
                stop <- w497 stop-if-true
                n268 = global read "Robot Global Data.vi" "What to do"() -> (w498:string)
                n269 = case shown="\"Turn Right\"" w498 {
                  tunnel: [FALSE FALSE FALSE FALSE TRUE] -> w497
                  frame "Far", Default {
                    n270 = call "Drive Forward.vi"("Time"=0.01, "Speed"=1.0) -> ()  [unwired: 9 in, 1 out]
                  }
                  frame "Wide" {
                  }
                  frame "Turn Left" {
                    n271 = call "Drive Turn.vi"("Time"=0.01, "Speed"=0.14, "Direction"=-1.0) -> ()  [unwired: 8 in, 1 out]
                  }
                  frame "Turn Right" {
                    n272 = call "Drive Turn.vi"("Time"=0.01, "Speed"=0.14, "Direction"=1.0) -> ()  [unwired: 8 in, 1 out]
                  }
                  frame "Good" {
                  }
                }
              }
              n273 = call "Stop.vi"("Time"=0.5, "error in"=w454) -> ("error out"=w453:errorcluster)  [unwired: 8 in, 1 out]
              n274 = while {
                tunnel: w453 -> [w480]
                tunnel: [w480] -> w451
                stop <- w481 stop-if-true
                n275 = global read "Robot Global Data.vi" "What to do"() -> (w482:string)
                n276 = case shown="\"Good\"" w482 {
                  tunnel: [FALSE FALSE FALSE FALSE TRUE] -> w481
                  frame "Far", Default {
                    n277 = call "Drive Forward.vi"("Time"=0.01, "Speed"=1.0) -> ()  [unwired: 9 in, 1 out]
                  }
                  frame "Wide" {
                  }
                  frame "Turn Left" {
                    n278 = call "Drive Turn.vi"("Time"=0.01, "Speed"=0.14, "Direction"=-1.0) -> ()  [unwired: 8 in, 1 out]
                  }
                  frame "Turn Right" {
                    n279 = call "Drive Turn.vi"("Time"=0.01, "Speed"=0.14, "Direction"=1.0) -> ()  [unwired: 8 in, 1 out]
                  }
                  frame "Good" {
                  }
                }
              }
              n280 = call "Stop.vi"("Time"=0.5, "error in"=w451) -> ("error out"=w450:errorcluster)  [unwired: 8 in, 1 out]
              n281 = while {
                tunnel: w450 -> [_]
                stop <- w457 stop-if-true
                n282 = global read "Robot Global Data.vi" "What to do"() -> (w458:string)
                n283 = case shown="\"Good\"" w458 {
                  tunnel: [FALSE FALSE FALSE FALSE w475] -> w457
                  frame "Far", Default {
                    n284 = call "Drive Forward.vi"("Time"=0.01, "Speed"=1.0) -> ()  [unwired: 9 in, 1 out]
                  }
                  frame "Wide" {
                  }
                  frame "Turn Left" {
                    n285 = call "Drive Turn.vi"("Time"=0.01, "Speed"=0.14, "Direction"=-1.0) -> ()  [unwired: 8 in, 1 out]
                  }
                  frame "Turn Right" {
                    n286 = call "Drive Turn.vi"("Time"=0.01, "Speed"=0.14, "Direction"=1.0) -> ()  [unwired: 8 in, 1 out]
                  }
                  frame "Good" {
                    n287 = call "Stop.vi"("Time"=0.5) -> ("error out"=w472:errorcluster)  [unwired: 9 in, 1 out]
                    n288 = local read "Speed"() -> (w471:dbl)
                    n289 = call "Shooting Shoot.vi"("Power"=w471, "error in (no error)"=w472) -> ("error out"=w473:errorcluster)  [unwired: 9 in]
                    n290 = call "Stop.vi"("Time"=0.5, "error in"=w473) -> ("error out"=w476:errorcluster)  [unwired: 8 in, 1 out]
                    n291 = case shown="No Error" w476 {
                      tunnel: [TRUE TRUE] -> w475
                      frame No Error {
                      }
                      frame Error {
                      }
                    }
                  }
                }
              }
            }
            frame True {
              # "PICNIC BASKET"
              # "PICNIC BASKET"
              # "PICNIC BASKET"
              # "PICNIC BASKET"
              n292 = local write "Stuck?"(w512) -> ()
            }
          }
        }
        frame 2 {
          # "Cross Defense"
          # "Stop .5 Secs"
          # "Fast Forward .5 Secs"
          # "Stop .5 Secs"
          # "Back Slow 2 Secs"
          # "Stop for .5 Secs"
          # "Go for 3 Secs"
          # "For the ones that are shove forward"
          n293 = call "Stop.vi"("Time"=0.1) -> ("error out"=w550:errorcluster)  [unwired: 9 in, 1 out]
          n294 = call "Drive Forward.vi"("Time"=1.3, "Speed"=1.0, "error in"=w550) -> ("error out"=w555:errorcluster)  [unwired: 8 in]
          n295 = call "Arm Auto.vi"("Time"=3.0, "U=T\nD=F"=FALSE ("U=T\nD=F"), "error in"=w550) -> ()  [unwired: 8 in, 1 out]
          n296 = call "Stop.vi"("Time"=0.5, "Stop Arm?"=FALSE, "error in"=w555) -> ()  [unwired: 7 in, 2 out]
          n297 = disable-structure shown="Disabled" {
            frame Disabled {
              n298 = local read "Position"() -> (w563:dbl)
              n299 = call "Drive Turn.vi"("Time"=0.25, "Speed"=1.0, "Direction"=w563) -> ("error out"=w561:errorcluster)  [unwired: 8 in]
              n300 = Not Equal?(x=w563, y=0.0) -> (x != y?=w560:bool)
              n301 = call "Stop.vi"("Time"=0.5, "Stop Arm?"=FALSE, "error in"=w561) -> ("error out"=w559:errorcluster)  [unwired: 7 in, 1 out]
              n302 = case shown="False" w560 {
                tunnel: w559 -> [w568 w572]
                tunnel: [w568 w569] -> w556
                frame False {
                }
                frame True {
                  n303 = call "Drive Forward.vi"("Time"=0.3, "Speed"=0.25, "error in"=w572) -> ("error out"=w569:errorcluster)  [unwired: 8 in]
                }
              }
              n304 = call "Stop.vi"("Time"=0.5, "Stop Arm?"=FALSE, "error in"=w556) -> ()  [unwired: 7 in, 2 out]
            }
            frame Enabled {
            }
          }
        }
        frame 3 {
          # "Up to Line"
          # "Stop for .5 Secs"
          # "Go for 3 Secs"
          # "For the ones that are shove forward"
          n305 = call "Drive Forward.vi"("Time"=0.5, "Speed"=1.0) -> ("error out"=w576:errorcluster)  [unwired: 9 in]
          n306 = call "Stop.vi"("Time"=0.5, "error in"=w576) -> ()  [unwired: 8 in, 2 out]
        }
        frame 0, Default {
          # "Disabled"
          n307 = call "Stop.vi"("Time"=0.5) -> ()  [unwired: 9 in, 2 out]
        }
      }
    }
    frame 8 {
      # "Low Bar"
      n308 = call "Stop.vi"("Time"=0.5) -> ()  [unwired: 9 in, 2 out]
    }
    frame 9 {
      # "Spy"
      n309 = case shown="2" w579 {
        frame 1 {
          # "Shoot"
          # "Perhaps add a go forward clause"
          n310 = call "Shoot.vi"("Time"=4.0, "Power Top Wheek"=-0.65 ("Power")) -> ("error out"=w583:errorcluster)  [unwired: 9 in]
          n311 = call "Indexing.vi"("TIme"=1.0, "Speed"=1.0, "error in"=w583) -> ("error out"=w582:errorcluster)  [unwired: 8 in]
          n312 = call "Stop.vi"("Time"=0.5, "error in"=w582) -> ()  [unwired: 8 in, 2 out]
        }
        frame 2 {
          # "Cross Defense"
          # "For the ones that are shove forward"
          n313 = call "Stop.vi"("Time"=0.5) -> ()  [unwired: 9 in, 2 out]
        }
        frame 3 {
          # "Up to Line"
          # "For the ones that are shove forward"
          n314 = call "Shoot.vi"("Time"=4.0, "Power Top Wheek"=-0.65 ("Power")) -> ("error out"=w602:errorcluster)  [unwired: 9 in]
          n315 = call "Indexing.vi"("TIme"=1.0, "Speed"=1.0, "error in"=w602) -> ("error out"=w601:errorcluster)  [unwired: 8 in]
          n316 = call "Stop.vi"("Time"=0.5, "error in"=w601) -> ("error out"=w599:errorcluster)  [unwired: 8 in, 1 out]
          n317 = call "Drive Turn.vi"("Time"=0.25, "Speed"=0.5, "Direction"=1.0, "error in"=w599) -> ("error out"=w595:errorcluster)  [unwired: 7 in]
          n318 = call "Stop.vi"("Time"=0.5, "error in"=w595) -> ("error out"=w590:errorcluster)  [unwired: 8 in, 1 out]
          n319 = call "Drive Forward.vi"("Time"=8.25, "Speed"=0.2, "error in"=w590) -> ("error out"=w594:errorcluster)  [unwired: 8 in]
          n320 = call "Stop.vi"("Time"=0.5, "error in"=w594) -> ()  [unwired: 8 in, 2 out]
        }
        frame 0, Default {
          # "Disabled"
          n321 = call "Stop.vi"("Time"=1.0) -> ()  [unwired: 9 in, 2 out]
        }
      }
    }
  }
  n322 = case shown="3" w8 {
    tunnel: [1.0 1.0 1.0 1.0 -1.0] -> w5
    tunnel: [-0.65 -0.65 -0.7 -0.7 -0.7] -> w1
    frame 0 {
      # "Far Left"
    }
    frame 1 {
      # "Left"
    }
    frame 2, Default {
      # "Middle"
    }
    frame 3 {
      # "Right"
    }
    frame 4 {
      # "Far Right"
    }
  }
  n323 = local write "Speed"(w1) -> ()
  n324 = local write "Position"(w5) -> ()
  "Stuck?" <- FALSE ("Stuck?")
